vi "configAO.vi"(8 "error in (no error)":errorcluster, 10 "Channels: AO":T1 {"AO f (Hz)" min=0.001 max=10000.0; "AO DC (V)" format="%.3p"; "AO Amp (V)" format="%.3p"}, 11 "Instrument.Lockin in":refnum<class "Instrument.Lockin.lvclass">) -> (0 "error out":errorcluster, 3 "Instrument.Lockin out":refnum<class "Instrument.Lockin.lvclass">)   [LabVIEW 2016, in "Instrument.Lockin.lvclass"]
doc: "API to configure AO.\n\nIf address=\"\", this API reads from localhost\nIf address is remote lockin, you need to add this computer to allowed whitelist on the lockin computer you are trying to access."
uses:
  Instrument.Lockin.lvclass
  LockinDAQ/Typedefs/AO-cluster.ctl
  LockinDAQ/Typedefs/AO_Amp-array.ctl
  LockinDAQ/Typedefs/AO_DC-array.ctl
  LockinDAQ/Typedefs/AO_f-array.ctl
  LockinDAQ/Typedefs/AO_phi-array.ctl
  LockinDAQ/Typedefs/Function-array.ctl
  LockinDAQ/Typedefs/Function-enum.ctl
  Typedefs/Instrument.Lockin.Commands--Enum.ctl
  LockinDAQ/LockinDAQ.lvclass
panel:
  # "1"
  # "2"
  # "3"
  # "4"
  # "5"
  # "6"
  # "7"
  # "8"
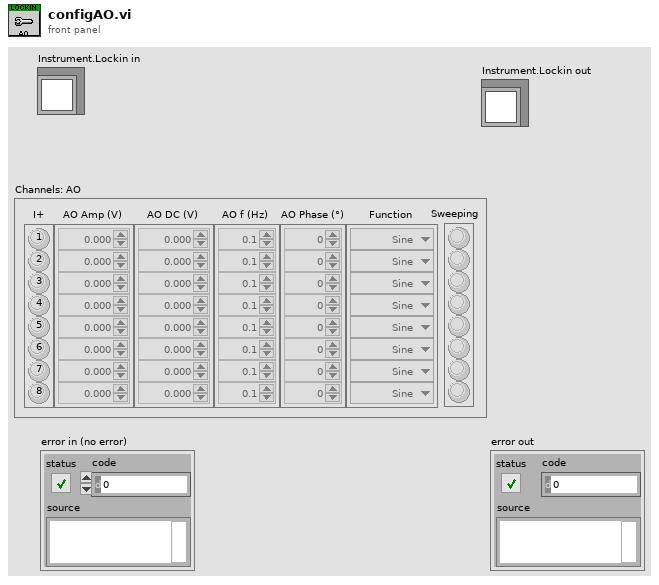
[diagram p1: front panel]
types:
  T1 = typedef "LockinDAQ.lvclass/AO-cluster.ctl" = cluster{"AO Amp (V)":T2, "AO DC (V)":T3, "AO f (Hz)":T4, "AO Phase (°)":T5, "Function":T6, "I+":bool[], "Sweeping":bool[]}
  T2 = typedef "LockinDAQ.lvclass/AO_Amp-array.ctl" = dbl[]
  T3 = typedef "LockinDAQ.lvclass/AO_DC-array.ctl" = dbl[]
  T4 = typedef "LockinDAQ.lvclass/AO_f-array.ctl" = dbl[]
  T5 = typedef "LockinDAQ.lvclass/AO_phi-array.ctl" = dbl[]
  T6 = typedef "LockinDAQ.lvclass/Function-array.ctl" = T7[]
  T7 = typedef "LockinDAQ.lvclass/Function-enum.ctl" = enum16{"Sine", "Triangle", "Square", "Sawtooth"}
  T8 = typedef "Instrument.Lockin.lvclass/Instrument.Lockin.Commands--Enum.ctl" = enum16{"configAO", "configAO_Amplitude", "configAO_DC", "configAO_Frequency", "configAO_Phase", "configAO_Function", "configAO_I+", "configREF", "configREF_Frequency", "configREF_Phase", "configREF_Filter", "configIVmode", "Reset", "configSampling", "Trigger", "getAO", "getAI", "getResults", "getTrigger", "getIVmode", "getSampling", "getAOconfig", "getREFconfig", "getREF_Filter", "configGain", "getGain", "configAutoSampling", "getAutoSampling", "configSweep"}
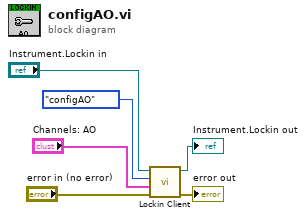
[diagram p0: block diagram]
diagram:
  n1 = call "Lockin Client.vi"("error in (no error)"="error in (no error)", "Data"="Channels: AO", "Command"=Instrument.Lockin.Commands--Enum."configAO", "Instrument.Lockin in"="Instrument.Lockin in") -> ("error out"=→"error out":errorcluster, "Instrument.Lockin out"=→"Instrument.Lockin out":refnum<class "Instrument.Lockin.lvclass">)  [unwired: 5 in, 1 out]
